vi "2015 Excavation.vi"(9 "Excavate?":bool, 10 "Winch angle":dbl format="%#_13g", 11 "Scoop angle":dbl format="%#_13g") -> (1 "Return Trip":bool, 2 "Winch PW":dbl format="%#_13g", 3 "Scoop PW":dbl format="%#_13g")   [LabVIEW 2014]
panel:
  out "Numeric":i32
  out "Exa Align":bool
  out "Last angle":dbl format="%#_13g"
  out "Exa comp":bool
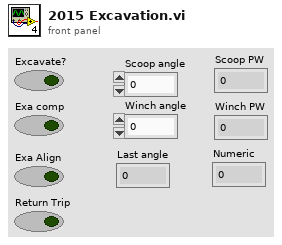
[diagram p1: front panel]
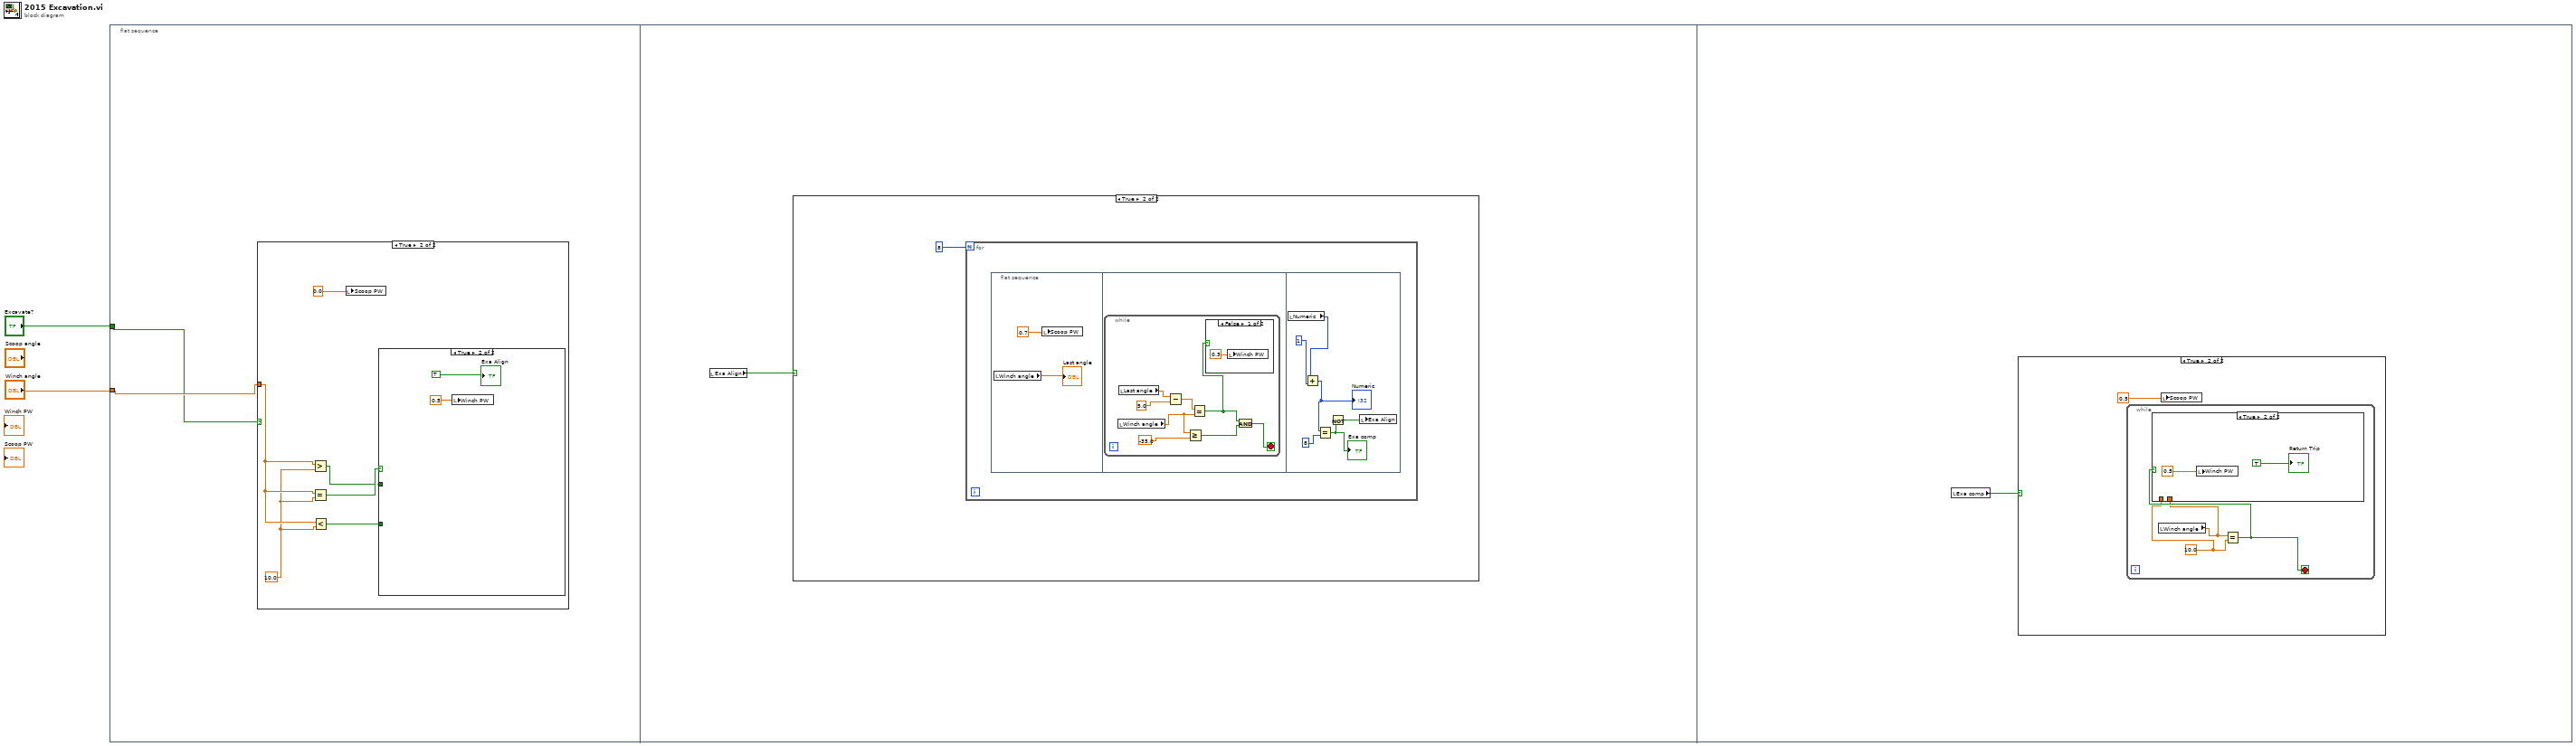
[diagram p0: block diagram]
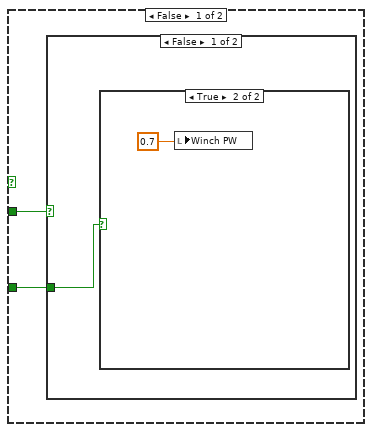
[diagram p3: hidden frame]
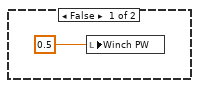
[diagram p4: hidden frame]
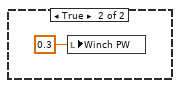
[diagram p5: hidden frame]
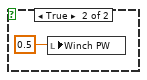
[diagram p7: hidden frame]
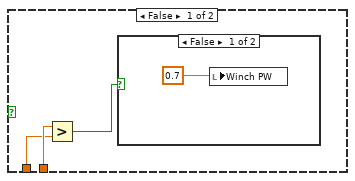
[diagram p9: hidden frame]
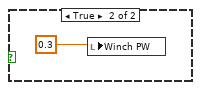
[diagram p10: hidden frame]
diagram:
  n1 = flat-sequence {
    tunnel: "Winch angle" -> [w4]
    tunnel: "Excavate?" -> [w3]
    frame #0 {
      n2 = case shown="True" w3 {
        tunnel: w4 -> [_ w10]
        frame False {
        }
        frame True {
          w9 = 10.0
          n3 = Greater?(x=w10, y=w9) -> (0:w7:bool)
          n4 = Equal?(x=w10, y=w9) -> (x = y?=w8:bool)
          n5 = Less?(x=w10, y=w9) -> (x < y?=w6:bool)
          n6 = local write "Scoop PW"(0.0) -> ()
          n7 = case shown="True" w8 {
            tunnel: w7 -> [w12 _]
            tunnel: w6 -> [w11 _]
            frame False {
              n8 = case shown="False" w12 {
                tunnel: w11 -> [w13 _]
                frame False {
                  n9 = case shown="True" w13 {
                    frame False {
                      n10 = local write "Winch PW"(0.5) -> ()
                    }
                    frame True {
                      n11 = local write "Winch PW"(0.7) -> ()
                    }
                  }
                }
                frame True {
                  n12 = local write "Winch PW"(0.3) -> ()
                }
              }
            }
            frame True {
              n13 = local write "Winch PW"(0.5) -> ()
              "Exa Align" <- TRUE
            }
          }
        }
      }
    }
    frame #1 {
      n14 = local read "Exa Align"() -> (w19:bool)
      n15 = case shown="True" w19 {
        frame False {
        }
        frame True {
          n16 = for {
            N: 8 -> [_]
            n17 = flat-sequence {
              frame #0 {
                n18 = local read "Winch angle"() -> (→"Last angle":dbl)
                n19 = local write "Scoop PW"(0.7) -> ()
              }
              frame #1 {
                n20 = while {
                  stop <- w23 stop-if-true
                  n21 = local read "Winch angle"() -> (w27:dbl)
                  n22 = local read "Last angle"() -> (w28:dbl)
                  n23 = Subtract(x=w28, y=5.0) -> (x-y=w30:dbl)
                  n24 = Greater Or Equal?(x=w27, y=-35.0) -> (x >= y?=w25:bool)
                  n25 = Equal?(x=w30, y=w27) -> (x = y?=w24:bool)
                  n26 = case shown="False" w24 {
                    frame False {
                      n27 = local write "Winch PW"(0.3) -> ()
                    }
                    frame True {
                      n28 = local write "Winch PW"(0.5) -> ()
                    }
                  }
                  n29 = And(x=w24, y=w25) -> (x .and. y?=w23:bool)
                }
              }
              frame #2 {
                n30 = local read "Numeric"() -> (w37:i32)
                n31 = Add(x=w37, y=1) -> (x+y=w33:i32)
                "Numeric" <- w33
                n32 = Equal?(x=w33, y=8) -> (x = y?=w34:bool)
                "Exa comp" <- w34
                n33 = Not(x=w34) -> (.not. x?=w35:bool)
                n34 = local write "Exa Align"(w35) -> ()
              }
            }
          }
        }
      }
    }
    frame #2 {
      n35 = local read "Exa comp"() -> (w39:bool)
      n36 = case shown="True" w39 {
        frame False {
        }
        frame True {
          n37 = while {
            stop <- w43 stop-if-true
            w41 = 10.0
            n38 = local read "Winch angle"() -> (w42:dbl)
            n39 = Equal?(x=w42, y=w41) -> (x = y?=w43:bool)
            n40 = case shown="True" w43 {
              tunnel: w42 -> [w46 _]
              tunnel: w41 -> [w45 _]
              frame False {
                n41 = Greater?(x=w46, y=w45) -> (0:w44:bool)
                n42 = case shown="False" w44 {
                  frame False {
                    n43 = local write "Winch PW"(0.7) -> ()
                  }
                  frame True {
                    n44 = local write "Winch PW"(0.3) -> ()
                  }
                }
              }
              frame True {
                n45 = local write "Winch PW"(0.5) -> ()
                "Return Trip" <- TRUE
              }
            }
          }
          n46 = local write "Scoop PW"(0.5) -> ()
        }
      }
    }
  }
